vi "Create Fast Tree Shortcuts.vi"(8 "error in":errorcluster, 11 "ParseGDSII in":refnum<class "ParseGDSII.lvclass">) -> (0 "error out":errorcluster, 3 "ParseGDSII out":refnum<class "ParseGDSII.lvclass">)   [LabVIEW 2019, in "ParseGDSII.lvclass"]
uses:
  ParseGDSII.lvclass
  ParseGDSII.lvclass/ParseGDSII.ctl
  Fast Tree/Fast Tree.lvclass
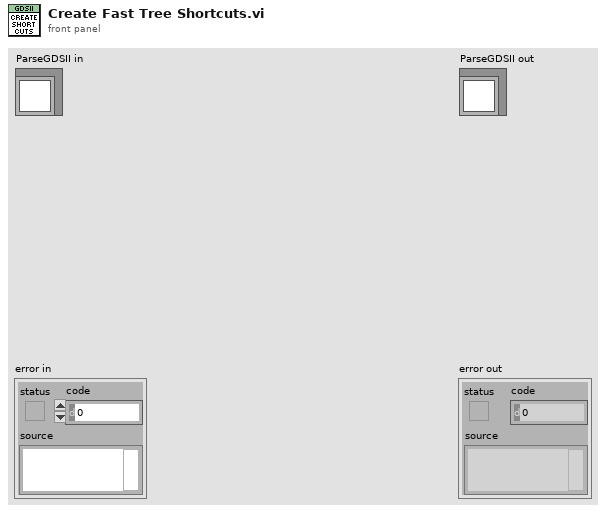
[diagram p1: front panel]
types:
  T1 = cluster{"Record Type":string, "Payload":string, "Parent Index":i32, "First Child Index":i32, "Next Sibling Index":i32}[]
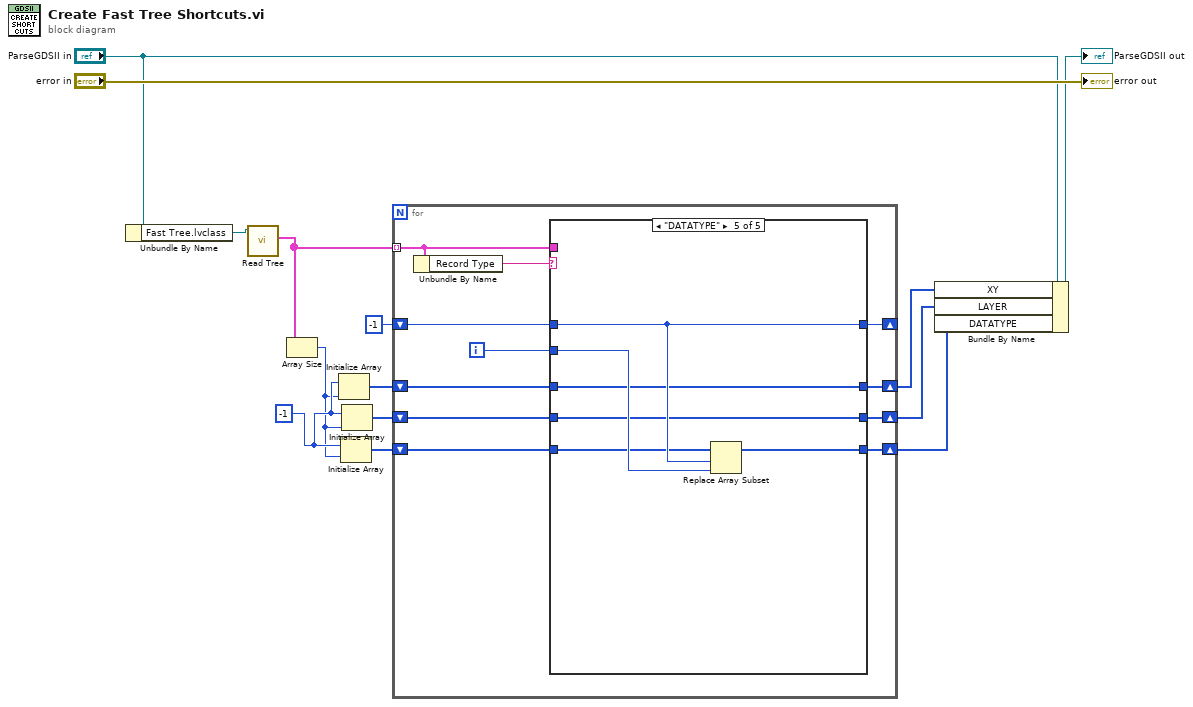
[diagram p0: block diagram]
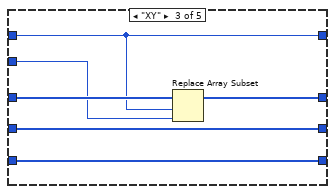
[diagram p4: hidden frame]
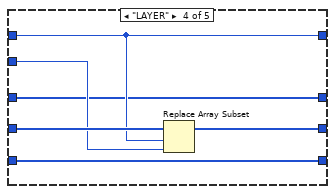
[diagram p5: hidden frame]
diagram:
  w9 = -1
  n1 = Unbundle By Name("ParseGDSII in") -> ("Fast Tree.lvclass"=w7:refnum<class "Fast Tree.lvclass">)
  n2 = call-dynamic "Read Tree.vi"("Fast Tree in"=w7) -> ("Tree"=w6:T1)  [unwired: 8 in, 2 out]
  n3 = Array Size(array=w6) -> (size(s)=w8:i32)
  n4 = Initialize Array(w9, w8) -> (w13:i32[])
  n5 = Initialize Array(w9, w8) -> (w10:i32[])
  n6 = Initialize Array(w9, w8) -> (w11:i32[])
  n7 = for {
    tunnel: w6 -> [w24] mode=indexing
    shift-right: [w22] -> w3
    shift-left: w13 -> [w23]
    shift-right: [w19] -> _
    shift-left: -1 -> [w21]
    shift-right: [w17] -> w2
    shift-left: w11 -> [w18]
    shift-right: [w15] -> w1
    shift-left: w10 -> [w16]
    i -> [w20]
    n8 = Unbundle By Name(w24) -> ("Record Type"=w25:string)
    n9 = case shown="\"DATATYPE\"" w25 {
      tunnel: w24 -> [_ _ _ _ _]
      tunnel: w23 -> [w29 w33 w38 w41 w49]
      tunnel: [w29 w33 w39 w41 w49] -> w22
      tunnel: w21 -> [w28 _ w35 w43 w51]
      tunnel: w20 -> [_ w32 w37 w42 w50]
      tunnel: [w28 w32 w35 w43 w51] -> w19
      tunnel: w18 -> [w27 w31 w36 w44 w46]
      tunnel: [w27 w31 w36 w45 w46] -> w17
      tunnel: w16 -> [w26 w30 w34 w40 w47]
      tunnel: [w26 w30 w34 w40 w48] -> w15
      frame Default {
      }
      frame "AREF", "BOUNDARY", "PATH", "SREF" {
      }
      frame "XY" {
        n10 = Replace Array Subset(array=w38, new element=w37, index=w35) -> (w39:i32[])
      }
      frame "LAYER" {
        n11 = Replace Array Subset(array=w44, new element=w42, index=w43) -> (w45:i32[])
      }
      frame "DATATYPE" {
        n12 = Replace Array Subset(array=w47, new element=w50, index=w51) -> (w48:i32[])
      }
    }
  }
  n13 = Bundle By Name(cluster="ParseGDSII in", "XY"=w3, "LAYER"=w2, "DATATYPE"=w1) -> (→"ParseGDSII out":refnum<class "ParseGDSII.lvclass">)
  "error out" <- "error in"
